vi "DLCpro example.vi"() -> ()   [LabVIEW 2013]
panel:
  out "Status":string
  in  "Password":string="Your password"
  in  "Scan Offset / V":dbl(knob)=29.8133088574562 scale=20.0..40.0
  in  "Scan Amp / V":dbl(knob)=65.1788930133066 scale=50.0..80.0
  out "XY-Graph":T1(graph)
  in  "connection":enum32{"TCP/IP", "USB"}(radio)
  in  "COM port":refnum<visa-resource-name>="COM1"
  in  "IP Address of DLC pro":string="192.168.1.200"
  out "Serial number":string
  in  "DeCof-command":string="(param-ref 'ul)"
  in  "stop":bool
  in  "send command":bool
  out "Answer string":string
  # "WARNING!\nConnecting to a DLC pro will alter its scan settings, including scan amplitude and scan offset by using the following parameters:\n-laser1:scan:enabled\n-laser1:scope:variant\n-laser1:scope:channelx:xy-signal\n-laser1:scope:channel1:signal\n-laser1:scan:amplitude \n-laser1:scan:offset\n\n1. Connecting to the DLC pro\n \na) Connection via TCP/IP\n\nWrite the IP Address of your DLC pro into the input field \"IP Address\" (e.g., 192.168.1.200).\n \nNOTE!\nThe DLC pro has to be connected to a local area network (LAN) or directly to a PC \n(e.g., with a cross link cable).  Further, the DLC pro and the PC must have the same \nsubnet mask and different IP addresses. You can edit these parameters of your\ndevice in the section \"Network Settings\" on your DLC pro. To connect the DLC pro \ndirectly to a computer, disable DHCP on both devices, set the same subnet mask \n(e.g., 255.255.255.0) and different IP addresses (e.g., 192.168.1.200 and 192.168.1.201)\n\n\nb) Connection via USB\n\nSelect the virtual COM port of your DLC pro in the field \"COM port\" (e.g., COM1).\n\nNOTE!\nFor DLC pro control via USB, the control computer must be connected to the USB connector at the MC/MC+ module via a micro USB cable with connector type B. Further, a specific USB driver has to be installed on your computer. When connecting your DLC pro to a USB port of your PC, it will be identified as a \"DLCpro\" device  and registered as a virtual COM port.\nDriver insatllation:\n- Make sure that the DLC pro is not connected with the control computer via  USB.  \n- You need two files for the installation of the driver which you find on your TOPTICA USB stick in the folder \"2_PC_GUI_...\". Their names are \"dlcpro-usb-serial.cat\" and \"dlcpro-usb-serial.inf\".\n- To install the driver, copy both files to the same location on your computer, right-click \n\"dlcpro-usb-serial.inf\", click \"install\", and confirm the installation in the dialog window.\n\n\n2. Start the program. If you can see the serial number of your DLC pro the connection was successful. If you have assigned a password for your device insert it to the field \"Password\". If you didn't assign a password you can ignore this field. The \"Status\" indicator should show \"READY\" now.\n\n3. Type arbitrary DeCof commands to the input field \"DeCof command\" and send them to the device by pushing the button \"SEND COMMAND\". At the output field \"Answer string\", you can see the device's answer.\n\nDeCof examples:\n\nThe value of a parameter can be retrieved with the param-ref instruction.  Its return value is the value of the parameter being queried. For example, to get the current user level, you have to type the following expression to the input field, where \"ul\" specifies the parameter  of the userlevel:\n\n(param-ref 'ul)\n\nTo change a parameter value, use the param-set! instruction.  Its return value is zero or\npositive integer in case of success and a negative number in case of an error. For example, to change the display brightness you have to type the following expression where display:brightness specifies the parameter of the brightness and 50 is the set value:\n\n(param-set! 'display:brightness 50)\n\nTo set the brightness back to it's maximum value, type:\n\n(param-set! 'display:brightness 100)\n\nTo execute a command use the exec instruction. For example, to play a melody with the DLC pro type:\n\n(exec 'buzzer:play \"A A A A A E E H E H E AAAA\")\n\nbuzzer:play is the command and  A A A A A E E H E H E AAAA is the argument of this command.\n\nOther parameters and commands can be looked up in the documentation (\"DLCpro-Command-Reference.pdf\").\n\n4. The graph shows an example how to retrieve data traces from the DLC pro device, in this case the \"PC Voltage\" and \"Scan Output\" traces. Watch the \"XY-Graph\" while changing the scan input parameters with the rotary knobs \"Scan Amp / V\" and  \"Scan Offset / V\".\n\n5. Stop the program and close the existing connection by pushing the \"STOP & CLOSE CONNECTION\" button."
  # "TOPTICA Photonics AG\n12.08.2015"
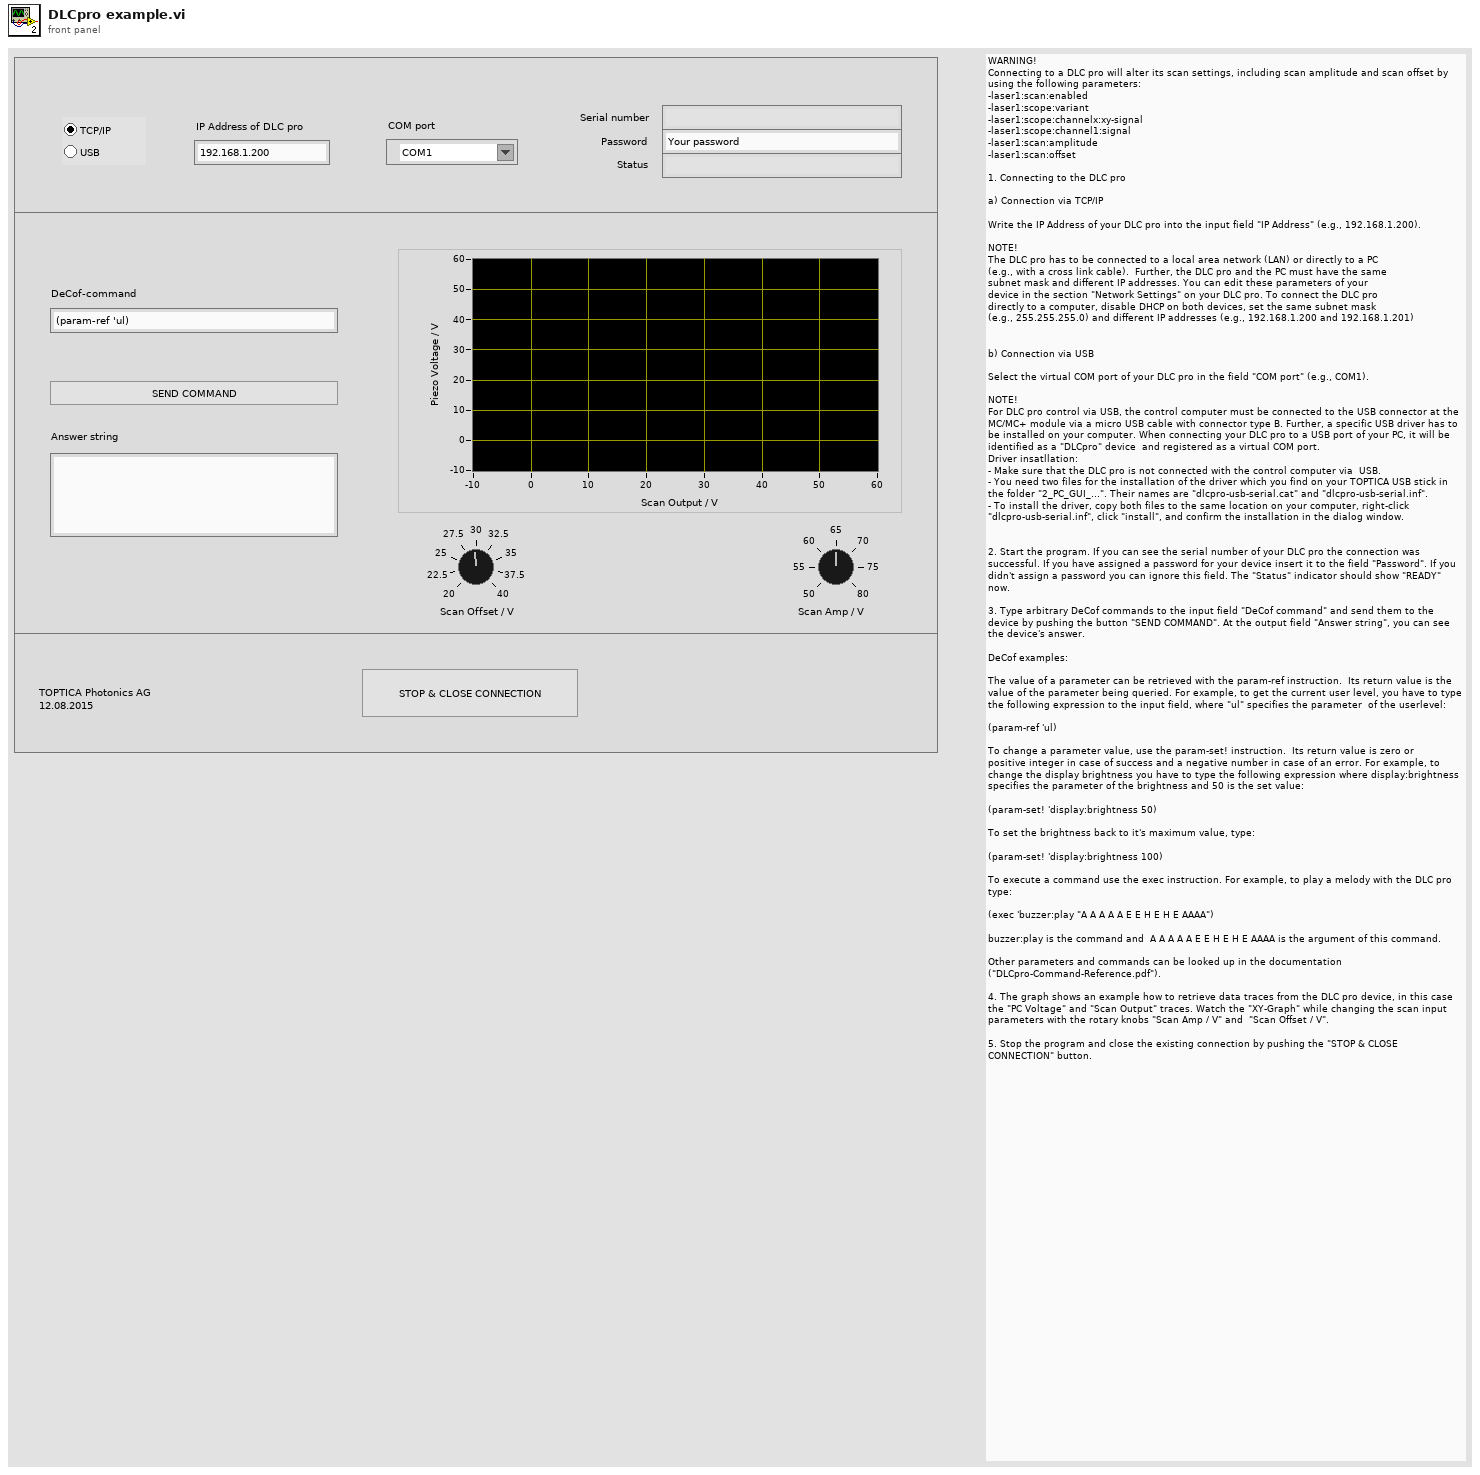
[diagram p1: front panel]
types:
  T1 = cluster{"Channel 1 data":sgl[], "Channel2 data":sgl[]}
  T2 = typedef "DeCoF connection.ctl" = cluster{"TCP/IP":bool, "VISA":refnum<visa-resource-name>, "TCP/IP ID":refnum<k5>}
  T3 = cluster{"float array":sgl[], "float array":sgl[]}
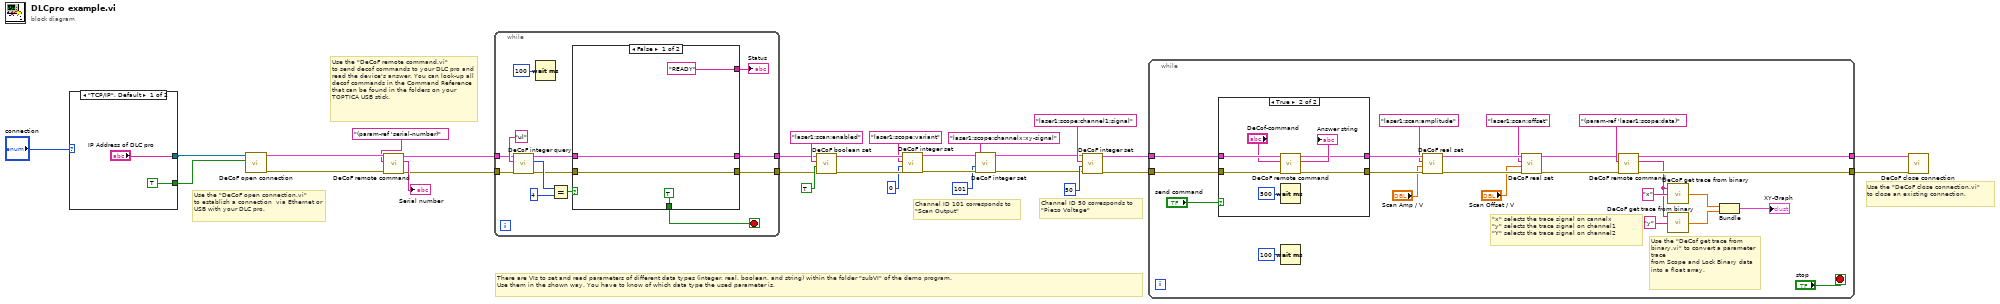
[diagram p0: block diagram]
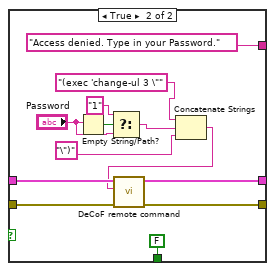
[diagram p2: hidden frame]
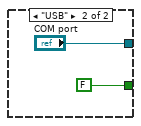
[diagram p3: hidden frame]
diagram:
  # "Channel ID 101 corresponds to\n\"Scan Output\""
  # "Channel ID 50 corresponds to\n\"Piezo Voltage\""
  # "There are VIs to set and read parameters of different data types (integer, real, boolean, and string) within the folder \"subVI\" of the demo program.\nUse them in the shown way. You have to know of which data type the used parameter is."
  # "Use the \"DeCoF remote command.vi\"\nto send decof commands to your DLC pro and read the device's answer. You can look-up all decof commands in the Command Reference that can be found in the folders on your TOPTICA USB stick."
  # "Use the \"DeCoF close connection.vi\"\nto close an existing connection."
  # "Use the \"DeCoF open connection.vi\"\nto establish a connection  via Ethernet or USB with your DLC pro."
  n1 = case shown="\"TCP/IP\", Default" "connection" {
    tunnel: ["IP Address of DLC pro" "COM port"] -> w24
    tunnel: [TRUE FALSE] -> w23
    frame "TCP/IP", Default {
    }
    frame "USB" {
    }
  }
  n2 = call "DeCoF open connection.vi"("TCP?"=w23, "address"=w24) -> ("error out"=w28:errorcluster, "Conncection ID out"=w29:T2)  [unwired: 4 in]
  n3 = call "DeCoF remote command.vi"("error in (no error)"=w28, "command"="(param-ref 'serial-number)", "Conncection ID in"=w29) -> ("error out"=w17:errorcluster, "answer string"=→"Serial number":string, "Conncection ID out"=w18:T2)  [unwired: 2 in, 2 out]
  n4 = while {
    tunnel: w18 -> [w38]
    tunnel: w17 -> [w37]
    tunnel: [w36] -> w16
    tunnel: [w35] -> w15
    stop <- w42 stop-if-true
    n5 = call "DeCoF integer query.vi"("error in"=w37, "param-name"="ul", "Conncection ID in"=w38) -> ("error out"=w40:errorcluster, "value"=w44:i32, "Conncection ID out"=w41:T2)  [unwired: 2 in]
    n6 = Wait (ms)(milliseconds to wait=u32 100) -> ()  [unwired: 1 out]
    n7 = Equal?(x=w44, y=4) -> (x = y?=w45:bool)
    n8 = case shown="False" w45 {
      tunnel: [TRUE FALSE] -> w42
      tunnel: w41 -> [w49 w62]
      tunnel: [w49 w61] -> w36
      tunnel: w40 -> [w48 w60]
      tunnel: [w48 w59] -> w35
      tunnel: ["READY" "Access denied. Type in your Password."] -> w39
      frame False {
      }
      frame True {
        n9 = Empty String/Path?(string/path="Password") -> (empty?=w54:bool)
        n10 = Select(t="1", s=w54, f="Password") -> (s? t:f=w51:string)
        n11 = Concatenate Strings("(exec 'change-ul 3 \"", w51, "\")") -> (w56:string)
        n12 = call "DeCoF remote command.vi"("error in (no error)"=w60, "command"=w56, "Conncection ID in"=w62) -> ("error out"=w59:errorcluster, "Conncection ID out"=w61:T2)  [unwired: 2 in, 3 out]
      }
    }
    "Status" <- w39
  }
  n13 = call "DeCoF boolean set.vi"("error in"=w15, "value"=TRUE, "param-name"="laser1:scan:enabled", "Conncection ID in"=w16) -> ("error out"=w9:errorcluster, "Conncection ID out"=w10:T2)  [unwired: 2 in]
  n14 = call "DeCoF integer set.vi"("error in"=w9, "value"=0, "param-name"="laser1:scope:variant", "Conncection ID in"=w10) -> ("error out"=w4:errorcluster, "Conncection ID out"=w6:T2)  [unwired: 2 in]
  n15 = call "DeCoF integer set.vi"("error in"=w4, "value"=101, "param-name"="laser1:scope:channelx:xy-signal", "Conncection ID in"=w6) -> ("error out"=w3:errorcluster, "Conncection ID out"=w5:T2)  [unwired: 2 in]
  n16 = call "DeCoF integer set.vi"("error in"=w3, "value"=50, "param-name"="laser1:scope:channel1:signal", "Conncection ID in"=w5) -> ("error out"=w11:errorcluster, "Conncection ID out"=w12:T2)  [unwired: 2 in]
  n17 = while {
    tunnel: w12 -> [w87]
    tunnel: w11 -> [w86]
    tunnel: [w82] -> w14
    tunnel: [w81] -> w13
    stop <- "stop" stop-if-true
    # "\"x\" selects the trace signal on cannelx\n\"y\" selects the trace signal on channel1\n\"Y\" selects the trace signal on channel2"
    # "Use the \"DeCof get trace from binary.vi\" to convert a parameter trace \nfrom Scope and Lock Binary data  into a float array."
    n18 = case shown="True" "send command" {
      tunnel: w87 -> [w89 w96]
      tunnel: w86 -> [w88 w95]
      tunnel: [w89 w92] -> w80
      tunnel: [w88 w91] -> w79
      frame False {
      }
      frame True {
        n19 = call "DeCoF remote command.vi"("error in (no error)"=w95, "command"="DeCof-command", "Conncection ID in"=w96) -> ("error out"=w91:errorcluster, "answer string"=→"Answer string":string, "Conncection ID out"=w92:T2)  [unwired: 2 in, 2 out]
        n20 = Wait (ms)(milliseconds to wait=u32 500) -> ()  [unwired: 1 out]
      }
    }
    n21 = Wait (ms)(milliseconds to wait=u32 100) -> ()  [unwired: 1 out]
    n22 = call "DeCoF real set.vi"("error in"=w79, "value"="Scan Amp / V", "param-name"="laser1:scan:amplitude" ("command"), "Conncection ID in"=w80) -> ("error out"=w68:errorcluster, "Conncection ID out"=w69:T2)  [unwired: 2 in]
    n23 = call "DeCoF real set.vi"("error in"=w68, "value"="Scan Offset / V", "param-name"="laser1:scan:offset" ("command"), "Conncection ID in"=w69) -> ("error out"=w77:errorcluster, "Conncection ID out"=w78:T2)  [unwired: 2 in]
    n24 = call "DeCoF remote command.vi"("error in (no error)"=w77, "command"="(param-ref 'laser1:scope:data)", "Conncection ID in"=w78) -> ("error out"=w81:errorcluster, "answer string"=w73:string, "Conncection ID out"=w82:T2)  [unwired: 2 in, 2 out]
    n25 = call "DeCoF get trace from binary.vi"("Block ID"="x" ("identifier 1"), "Binary in"=w73) -> ("float array"=w74:sgl[])  [unwired: 1 in]
    n26 = call "DeCoF get trace from binary.vi"("Block ID"="y", "Binary in"=w73) -> ("float array"=w71:sgl[])  [unwired: 1 in]
    n27 = Bundle("float array"=w74, "float array"=w71) -> (→"XY-Graph":T3)  [unwired: 1 in]
  }
  n28 = call "DeCoF close connection.vi"("error in (no error)"=w13, "Connection ID in"=w14) -> ()  [unwired: 4 in, 2 out]
